vi "Validate Parameters.vi"(8 "error in (no error)":errorcluster, 9 "Npts":i32, 10 "Fs (Hz)":dbl, 11 "Gate in":refnum<class "Gate.lvclass">) -> (0 "error out":errorcluster, 3 "Gate out":refnum<class "Gate.lvclass">)   [LabVIEW 2020, in "Gate.lvclass"]
uses:
  Gate.lvclass
  Gate.lvclass/Gate.ctl
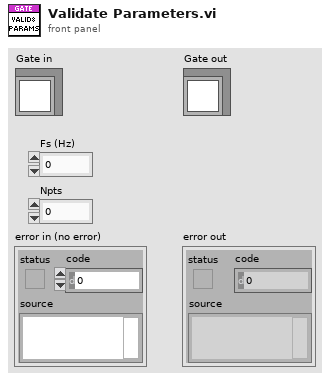
[diagram p1: front panel]
types:
  T1 = typedef "Gate.lvclass/Shape.ctl" = enum16{"OFF", "Rectangle", "Sine-squared", "Trapezoid"}
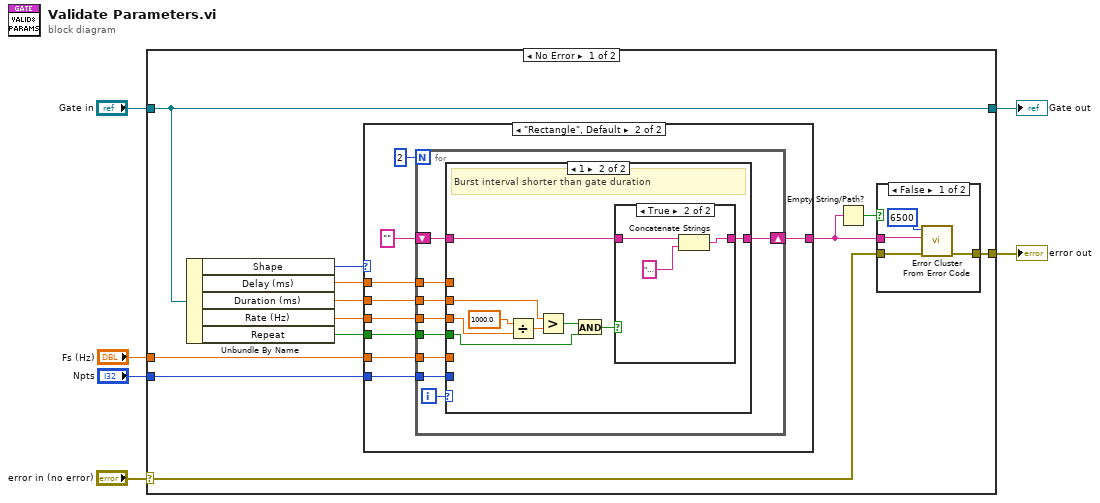
[diagram p0: block diagram]
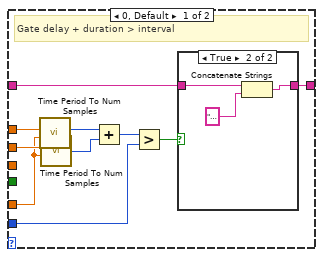
[diagram p4: hidden frame]
diagram:
  n1 = case shown="No Error" "error in (no error)" {
    selector: "error in (no error)" -> [w9 w70]
    tunnel: [w10 w70] -> w5
    tunnel: [w18 w69] -> w3
    tunnel: "Gate in" -> [w18 w69]
    tunnel: "Fs (Hz)" -> [w13 _]
    tunnel: "Npts" -> [w7 _]
    frame No Error {
      n2 = Unbundle By Name(w18) -> ("Shape"=w17:T1, "Delay (ms)"=w16:dbl, "Duration (ms)"=w15:dbl, "Rate (Hz)"=w14:dbl, "Repeat"=w8:bool)
      n3 = case shown="\"Rectangle\", Default" w17 {
        tunnel: w16 -> [_ w32]
        tunnel: w15 -> [_ w31]
        tunnel: w14 -> [_ w26]
        tunnel: w13 -> [_ w30]
        tunnel: [_ w27] -> w12
        tunnel: w8 -> [_ w25]
        tunnel: w7 -> [_ w24]
        frame "OFF" {
        }
        frame "Rectangle", Default {
          n4 = for {
            N: 2 -> [_]
            tunnel: w32 -> [w41]
            tunnel: w31 -> [w40]
            tunnel: w30 -> [w39]
            shift-right: [w37] -> w27
            shift-left: "" -> [w36]
            tunnel: w26 -> [w35]
            tunnel: w25 -> [w34]
            tunnel: w24 -> [w33]
            i -> [w38]
            n5 = case shown="1" w38 {
              tunnel: w41 -> [w51 _]
              tunnel: w40 -> [w45 w59]
              tunnel: w39 -> [w43 _]
              tunnel: [w48 w63] -> w37
              tunnel: w36 -> [w49 w64]
              tunnel: w35 -> [_ w62]
              tunnel: w34 -> [_ w57]
              tunnel: w33 -> [w42 _]
              frame 0, Default {
                # "Gate delay + duration > interval"
                n6 = call "Time Period To Num Samples.vi"("Duration (ms)"=w51, "Sampling rate (Hz)"=w43) -> ("Samples"=w46:i32)  [unwired: 5 in]
                n7 = call "Time Period To Num Samples.vi"("Duration (ms)"=w45, "Sampling rate (Hz)"=w43) -> ("Samples"=w44:i32)  [unwired: 5 in]
                n8 = Add(x=w46, y=w44) -> (x+y=w47:i32)
                n9 = Greater?(x=w47, y=w42) -> (0:w50:bool)
                n10 = case shown="True" w50 {
                  tunnel: w49 -> [w52 w54]
                  tunnel: [w52 w55] -> w48
                  frame False {
                  }
                  frame True {
                    n11 = Concatenate Strings(w54, "Gate (delay + duration) is wider than the interstimulus interval\n") -> (w55:string)
                  }
                }
              }
              frame 1 {
                # "Burst interval shorter than gate duration"
                n12 = Divide(x=1000.0, y=w62) -> (x/y=w60:dbl)
                n13 = Greater?(x=w59, y=w60) -> (0:w58:bool)
                n14 = And(x=w58, y=w57) -> (x .and. y?=w56:bool)
                n15 = case shown="True" w56 {
                  tunnel: w64 -> [w65 w67]
                  tunnel: [w65 w68] -> w63
                  frame False {
                  }
                  frame True {
                    n16 = Concatenate Strings(w67, "Gate is wider than burst interval") -> (w68:string)
                  }
                }
              }
            }
          }
        }
      }
      n17 = Empty String/Path?(string/path=w12) -> (empty?=w11:bool)
      n18 = case shown="False" w11 {
        tunnel: w12 -> [w22 _]
        tunnel: [w20 w23] -> w10
        tunnel: w9 -> [w19 w23]
        frame False {
          n19 = call <vilib>:"Error Cluster From Error Code.vi"("error in (no error)"=w19, "error message (\"\")"=w22, "error code (0)"=6500) -> ("error out"=w20:errorcluster)  [unwired: 6 in]
        }
        frame True {
        }
      }
    }
    frame Error {
    }
  }
  "error out" <- w5
  "Gate out" <- w3
